vi "Read DomeCommunicator.vi"(8 "error in (no error)":errorcluster, 11 "DomeController in":refnum<class "DomeController.lvclass">) -> (0 "error out":errorcluster, 2 "DomeCommunicator.lvclass":refnum<class "ATDomeCommunicator.lvclass">, 3 "DomeController out":refnum<class "DomeController.lvclass">)   [LabVIEW 2016, in "DomeController.lvclass"]
uses:
  DomeController.lvclass
  domeCommunicator/ATDomeCommunicator.lvclass
  DomeController.lvclass/DomeController.ctl
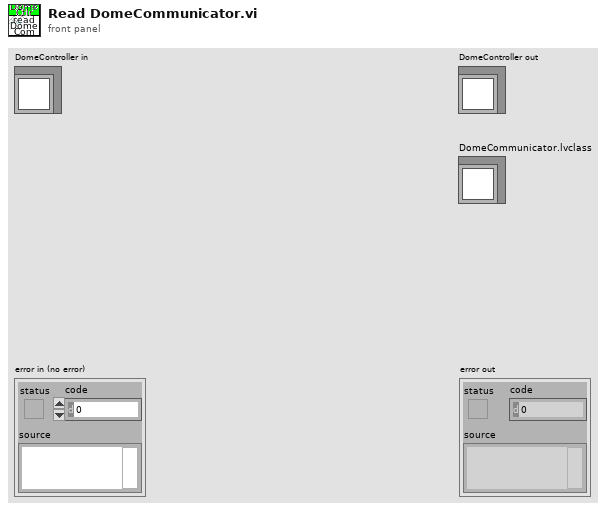
[diagram p1: front panel]
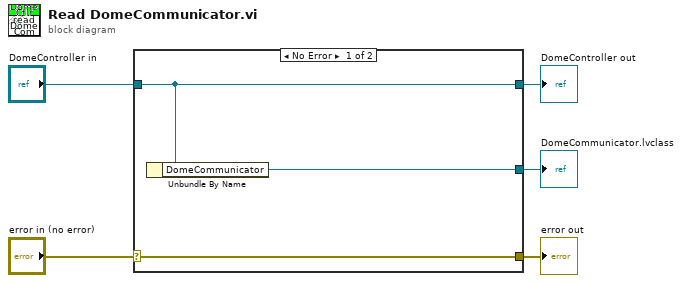
[diagram p0: block diagram]
diagram:
  n1 = case shown="No Error" "error in (no error)" {
    selector: "error in (no error)" -> [w8 w9]
    tunnel: [w8 w9] -> w4
    tunnel: [w7 w10] -> w2
    tunnel: "DomeController in" -> [w7 w10]
    tunnel: [w6 _] -> w1
    frame No Error {
      n2 = Unbundle By Name(w7) -> ("DomeCommunicator"=w6:refnum<class "ATDomeCommunicator.lvclass">)
    }
    frame Error {
    }
  }
  "error out" <- w4
  "DomeController out" <- w2
  "DomeCommunicator.lvclass" <- w1
